vi "smartHome-Old-Controllers.vi"(5 "Device in":refnum<k24>) -> (2 "Device out":refnum<k24>)   [LabVIEW 2014]
doc: "André Romero - 2017\nandretec@ifsc.usp.br"
uses:
  C:/user-Lab/AndreTec/GITs/andretec/Thorlabs-Vector-Move/kinesisTec/Kinesis/Thorlabs.MotionControl.TCube.DCServoCLI.dll
  kinesisTec/Kinesis/Thorlabs.MotionControl.TCube.DCServoCLI.dll
panel:
  out "array 2":bool[](array[boolean])
  out "array":bool[](array[boolean])
  out "String":string
  out "GetPOS 2":dbl
  out "GetPOS":dbl
  out "new Target":dbl
  out "old Target":dbl
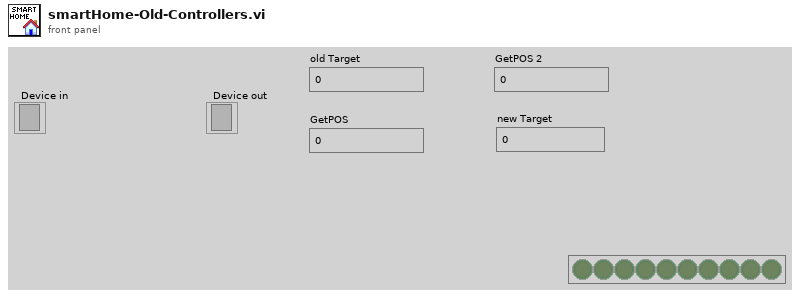
[diagram p1: front panel]
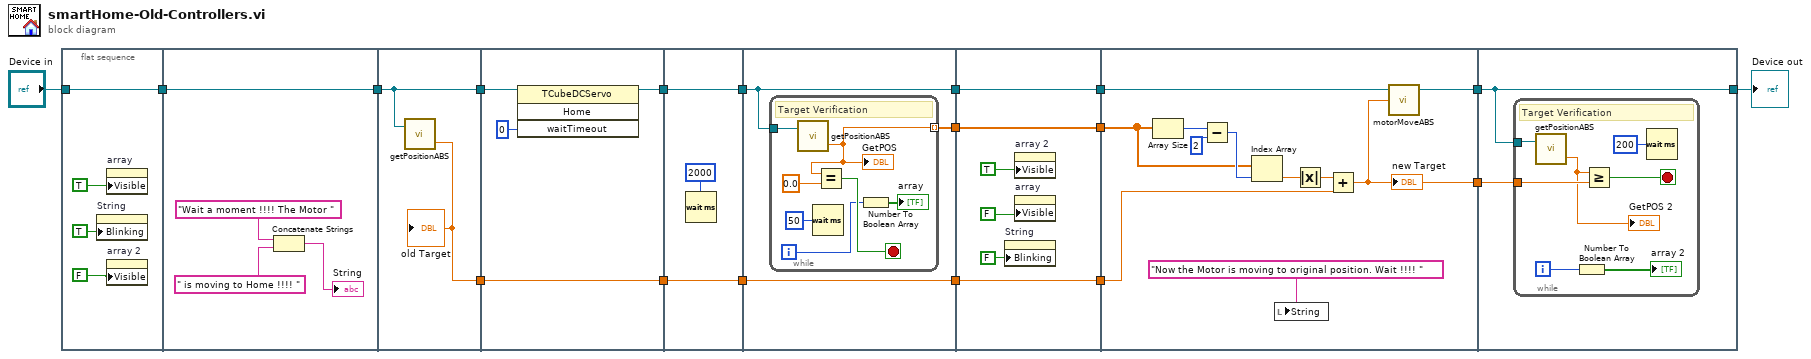
[diagram p0: block diagram]
diagram:
  n1 = flat-sequence {
    tunnel: "Device in" -> [w22]
    tunnel: [w22] -> w1
    tunnel: [w24] -> w8
    tunnel: w1 -> [w24]
    tunnel: [w28] -> w18
    tunnel: [w27] -> w17
    tunnel: w8 -> [w28]
    tunnel: [w31] -> w16
    tunnel: w18 -> [w30]
    tunnel: [w29] -> w15
    tunnel: w17 -> [w29]
    tunnel: [w35] -> w14
    tunnel: w16 -> [w35]
    tunnel: [w33] -> w13
    tunnel: w15 -> [w33]
    tunnel: w14 -> [w37]
    tunnel: [w38] -> w7
    tunnel: [w37] -> w5
    tunnel: w13 -> [w36]
    tunnel: [w36] -> w3
    tunnel: w7 -> [w51]
    tunnel: [w51] -> w6
    tunnel: w5 -> [w50]
    tunnel: [w50] -> w4
    tunnel: w3 -> [w49]
    tunnel: [w49] -> w2
    tunnel: w6 -> [w57]
    tunnel: w4 -> [w55]
    tunnel: w2 -> [w54]
    tunnel: [w56] -> w12
    tunnel: [w53] -> w11
    tunnel: [w64] -> w9
    tunnel: w12 -> [w64]
    tunnel: w11 -> [w63]
    frame #0 {
      n2 = property on="String" class="Str"("Blinking"=TRUE) -> ()  [unwired: 2 in, 2 out]
      n3 = property on="array" class="Arr (strict)"("Visible"=TRUE) -> ()  [unwired: 2 in, 2 out]
      n4 = property on="array 2" class="Arr (strict)"("Visible"=FALSE) -> ()  [unwired: 2 in, 2 out]
    }
    frame #1 {
      n5 = Concatenate Strings("Wait a moment !!!! The Motor ", " is moving to Home !!!! ") -> (→"String":string)
    }
    frame #2 {
      n6 = call "getPositionABS.vi"("Device"=w28) -> ("GetPOS"=w27:dbl)  [unwired: 1 in, 1 out]
      "old Target" <- w27
    }
    frame #3 {
      n7 = invoke class="TCubeDCServo" method="Home"(reference=w30, "waitTimeout"=0) -> (reference out=w31:refnum<k24>)  [unwired: 2 in, 3 out]
    }
    frame #4 {
      n8 = Wait (ms)(milliseconds to wait=u32 2000) -> ()  [unwired: 1 out]
    }
    frame #5 {
      n9 = while {
        tunnel: w37 -> [w45]
        tunnel: [w39] -> w38 mode=indexing
        i -> [w40]
        stop <- w42 stop-if-true
        # "Target Verification"
        n10 = call "getPositionABS.vi"("Device"=w45) -> ("GetPOS"=w39:dbl)  [unwired: 1 in, 1 out]
        "GetPOS" <- w39
        n11 = Wait (ms)(milliseconds to wait=u32 50) -> ()  [unwired: 1 out]
        n12 = Equal?(x=w39, y=0.0) -> (x = y?=w42:bool)
        n13 = Number To Boolean Array(number=w40) -> (Boolean array=→"array":bool[])
      }
    }
    frame #6 {
      n14 = property on="String" class="Str"("Blinking"=FALSE) -> ()  [unwired: 2 in, 2 out]
      n15 = property on="array 2" class="Arr (strict)"("Visible"=TRUE) -> ()  [unwired: 2 in, 2 out]
      n16 = property on="array" class="Arr (strict)"("Visible"=FALSE) -> ()  [unwired: 2 in, 2 out]
    }
    frame #7 {
      n17 = Array Size(array=w57) -> (size(s)=w60:i32)
      n18 = Subtract(x=w60, y=2) -> (x-y=w59:i32)
      n19 = Index Array(array=w57, index=w59) -> (element=w61:dbl)
      n20 = local write "String"("Now the Motor is moving to original position. Wait !!!! ") -> ()
      n21 = Absolute Value(x=w61) -> (abs(x)=w62:dbl)
      n22 = Add(x=w62, y=w54) -> (x+y=w53:dbl)
      "new Target" <- w53
      n23 = call "motorMoveABS.vi"("position"=w53, "Device in"=w55) -> ("Device out"=w56:refnum<k24>)  [unwired: 3 in]
    }
    frame #8 {
      n24 = while {
        tunnel: w64 -> [w70]
        tunnel: w63 -> [w69]
        i -> [w67]
        stop <- w68 stop-if-true
        # "Target Verification"
        n25 = call "getPositionABS.vi"("Device"=w70) -> ("GetPOS"=w65:dbl)  [unwired: 1 in, 1 out]
        "GetPOS 2" <- w65
        n26 = Number To Boolean Array(number=w67) -> (Boolean array=→"array 2":bool[])
        n27 = Greater Or Equal?(x=w65, y=w69) -> (x >= y?=w68:bool)
        n28 = Wait (ms)(milliseconds to wait=u32 200) -> ()  [unwired: 1 out]
      }
    }
  }
  "Device out" <- w9
